vi "Upload_File_S3.vi"(8 "error in (no error)":errorcluster, 11 "File_path":path) -> (0 "error out":errorcluster)   [LabVIEW 2018, in "TestStand_Control.lvlib"]
uses:
  TestStand_Control/TestStand_Control.lvlib
  <vilib>/AWS Toolkit/S3/PUT Object Request Parameters.ctl
  <vilib>/AWS Toolkit/S3/ACL.ctl
  <vilib>/AWS Toolkit/S3/Storage Class.ctl
  <vilib>/AWS Toolkit/Core/HTTP Request/Name Value Pair.ctl
  <vilib>/AWS Toolkit/Core/HTTP Request/AWS Credentials.ctl
  <vilib>/AWS Toolkit/S3/Bucket/Bucket.lvclass
  <vilib>/AWS Toolkit/Core/HTTP Request/HTTP Request.lvclass
  <vilib>/AWS Toolkit/S3/NI_AWS_S3.lvlib
panel:
  in  "Bucket name":string="vtaf-test-sample"
  in  "Object Parameters":T1={"Content Type"="text/html", "ACL"=enum."public-read", "Storage Class"=enum."STANDARD", "User-Defined Metadata"=[]}
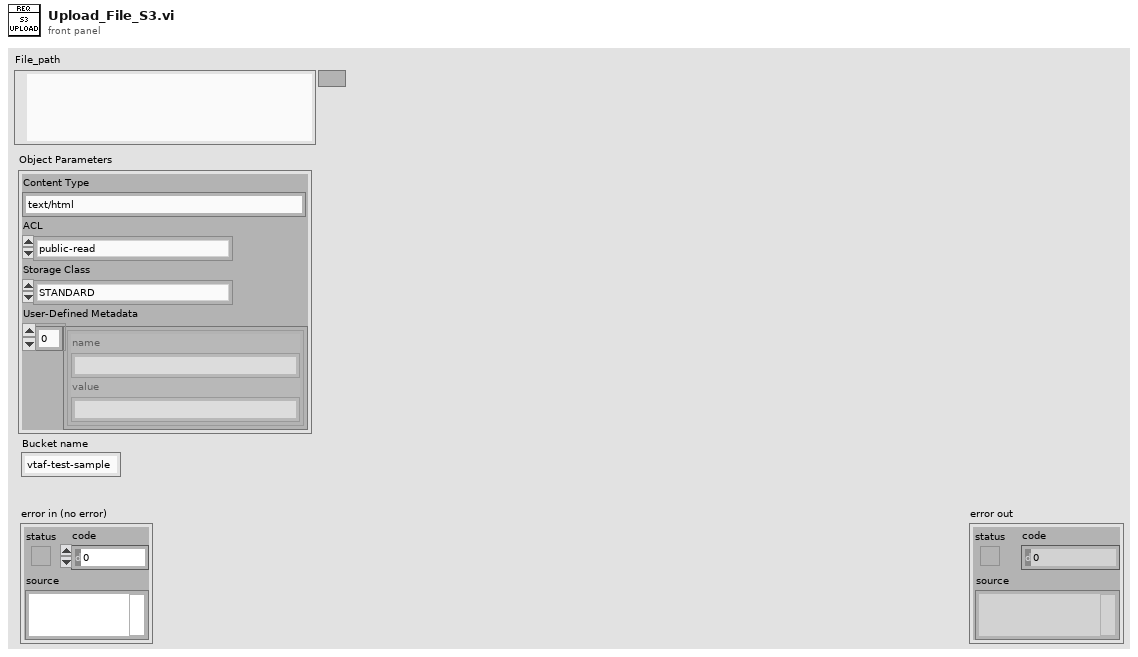
[diagram p1: front panel]
types:
  T1 = typedef "NI_AWS_S3.lvlib/PUT Object Request Parameters.ctl" = cluster{"Content Type":string, "ACL":T2, "Storage Class":T3, "User-Defined Metadata":T4[]}
  T2 = typedef "NI_AWS_S3.lvlib/ACL.ctl" = enum16{"private", "public-read", "public-read-write", "aws-exec-read", "authenticated-read", "bucket-owner-read", "bucket-owner-full-control"}
  T3 = typedef "NI_AWS_S3.lvlib/Storage Class.ctl" = enum16{"STANDARD", "REDUCED_REDUNDANCY"}
  T4 = typedef "NI_AWS_Core.lvlib/HTTP Request.lvclass/Name Value Pair.ctl" = cluster{"name":string, "value":string}
  T5 = typedef "NI_AWS_Core.lvlib/HTTP Request.lvclass/AWS Credentials.ctl" = cluster{"Access Key":string, "Secret Key":string}
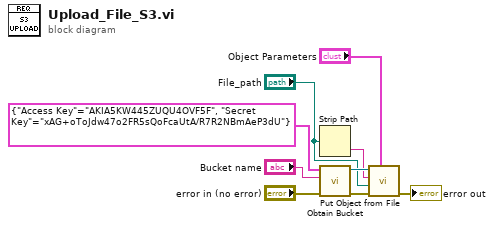
[diagram p0: block diagram]
diagram:
  n1 = Strip Path(path="File_path") -> (name=w4:string)  [unwired: 1 out]
  n2 = call <vilib>:"Obtain Bucket.vi"("error in (no error)"="error in (no error)", "Bucket name"="Bucket name", "AWS Credentials"=T5 {"Access Key"="AKIA5KW445ZUQU4OVF5F", "Secret Key"="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"}) -> ("error out"=w6:errorcluster, "Bucket"=w7:refnum<class "Bucket.lvclass">)  [unwired: 7 in]
  n3 = call <vilib>:"Put Object from File.vi"("Object Parameters"="Object Parameters", "error in (no error)"=w6, "File"="File_path", "Object Path"=w4, "Bucket in"=w7) -> ("error out"=→"error out":errorcluster)  [unwired: 2 in, 4 out]
